vi "MC.GetConfiguration.vi"(8 "error in (no error)":errorcluster, 11 "MC":refnum<class "MC.lvclass">) -> (0 "error out":errorcluster, 2 "Configuration":T1, 3 "MC out":refnum<class "MC.lvclass">)   [LabVIEW 2017, in "MC.lvclass"]
doc: "---------------------------------------------------------------\nJKI State Machine Objects™\nhttp://jki.net/state-machine-objects/\nCopyright (C) 2005-2015, JKI <info@jki.net>\nALL RIGHTS RESERVEDJKI State Machine Objects (SMO) 1.0.0.5\nJKI - JKI\nCopyright (c) 2016, JKI"
uses:
  MC.lvclass
  Typedefs/Configuration--Cluster.ctl
  MC.lvclass/MC.ctl
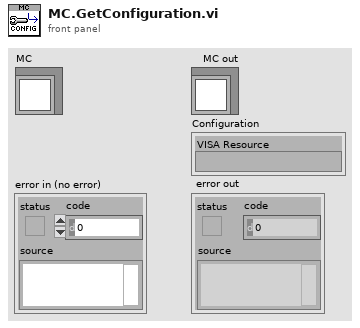
[diagram p1: front panel]
types:
  T1 = typedef "MC.lvclass/Configuration--Cluster.ctl" = cluster{"VISA Resource":string}
  T2 = typedef "MC.lvclass/PrivateData--Ref.ctl" = refnum<data-value>
  T3 = typedef "MC.lvclass/PrivateData--Cluster.ctl" = cluster{"Private Events":T4, "Configuration":T1}
  T4 = typedef "MC.lvclass/PrivateEvents--Cluster.ctl" = cluster{"SetWavelength":refnum<user-event>}
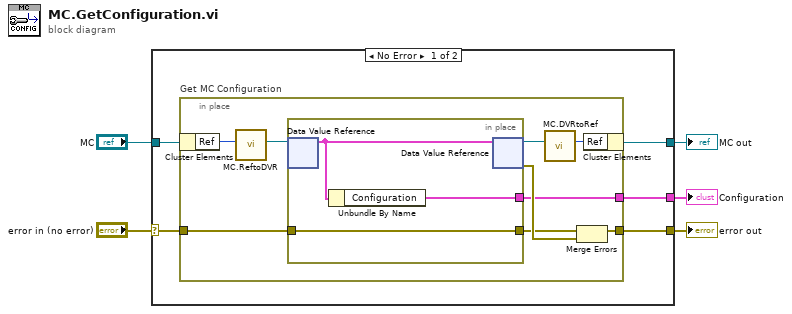
[diagram p0: block diagram]
diagram:
  n1 = case shown="No Error" "error in (no error)" {
    selector: "error in (no error)" -> [w9 w23]
    tunnel: "MC" -> [w10 w24]
    tunnel: [w8 w23] -> w4
    tunnel: [w7 w24] -> w3
    tunnel: [w6 _] -> w1
    frame No Error {
      n2 = in-place "Get MC Configuration" {
        in-place-border: w9 -> [w19]
        in-place-border: [w16] -> w8
        in-place-border: [w15] -> w6
        n3 = in-place-cluster #1(w10) -> ("Ref"=w12:u32)
        n4 = call "MC.ReftoDVR.vi"("Ref"=w12) -> ("Ref"=w11:T2)  [unwired: 10 in]
        n5 = in-place {
          in-place-border: w19 -> [w21]
          in-place-border: [w21] -> w17
          in-place-border: [w20] -> w15
          n6 = in-place-dvr #2(w11) -> (w22:T3)  [unwired: 1 out]
          n7 = Unbundle By Name(w22) -> ("Configuration"=w20:T1)
          n8 = in-place-dvr #2(w22) -> (w14:T2, w18:errorcluster)
        }
        n9 = call "MC.DVRtoRef.vi"("Ref"=w14) -> ("Ref"=w13:u32)  [unwired: 10 in]
        n10 = Merge Errors(w17, w18) -> (w16:errorcluster)
        n11 = in-place-cluster #1("Ref"=w13) -> (w7:refnum<class "MC.lvclass">)
      }
    }
    frame Error {
    }
  }
  "error out" <- w4
  "MC out" <- w3
  "Configuration" <- w1
